vi "Translate Coords to Grid.vi"(11 "Obstacle Avoidance Data":T1) -> (2 "Translation Vector":cluster{"X":dbl, "Y":dbl}, 3 "Obstacle Avoidance Data":T1)   [LabVIEW 2017]
panel:
  out "XY Graph":cluster{"X":dbl, "Y":dbl}[](graph)
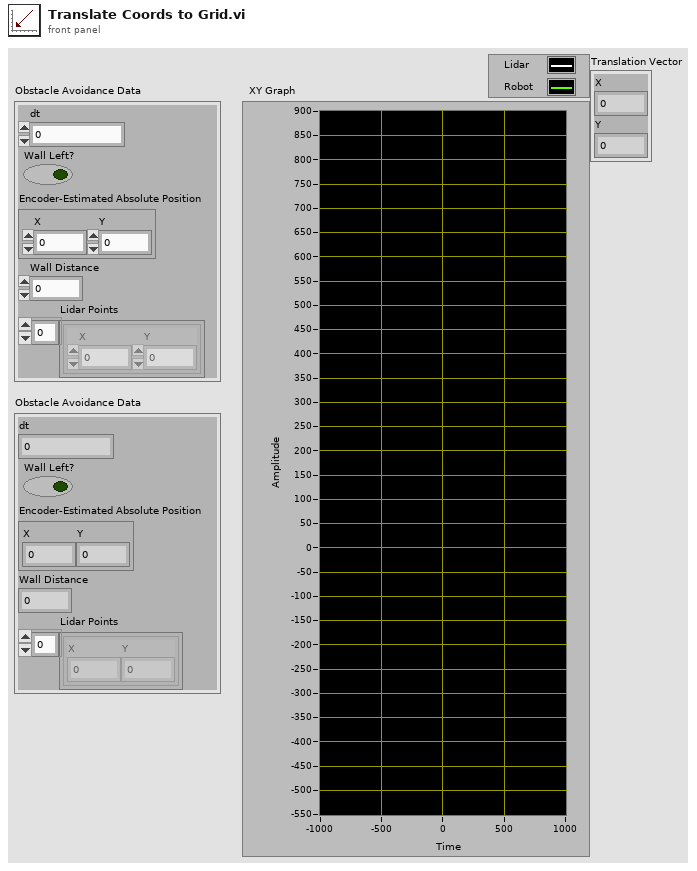
[diagram p1: front panel]
types:
  T1 = cluster{"dt":dbl, "Wall Left?":bool, "Encoder-Estimated Absolute Position":cluster{"X":dbl, "Y":dbl}, "Wall Distance":dbl, "Lidar Points":cluster{"X":dbl, "Y":dbl}[]}
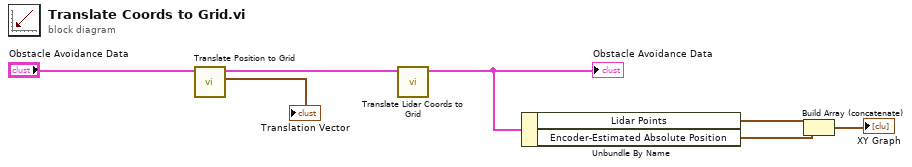
[diagram p0: block diagram]
diagram:
  n1 = call "Translate Position to Grid.vi"("Obstacle Avoidance Data"="Obstacle Avoidance Data") -> ("Translation Vector"=→"Translation Vector":cluster{"X":dbl, "Y":dbl}, "Obstactle Avoidance Data"=w6:T1)  [unwired: 9 in]
  n2 = call "Translate Lidar Coords to Grid.vi"("Obstacle Avoidance Data"=w6) -> ("Obstacle Avoidance Data"=w5:T1)  [unwired: 10 in]
  "Obstacle Avoidance Data" <- w5
  n3 = Unbundle By Name(w5) -> ("Lidar Points"=w4:cluster{"X":dbl, "Y":dbl}[], "Encoder-Estimated Absolute Position"=w3:cluster{"X":dbl, "Y":dbl})
  n4 = Build Array (concatenate)(w4, w3) -> (→"XY Graph":cluster{"X":dbl, "Y":dbl}[])
